vi "Factory.vi"(8 "error in":errorcluster, 10 "Class name":string) -> (0 "error out":errorcluster, 3 "Read Config out":refnum<class "Read Config File.lvclass">)   [LabVIEW 2025, in "Config Library.lvlib" / "Read Config File.lvclass"]
uses:
  Read Config File.lvclass
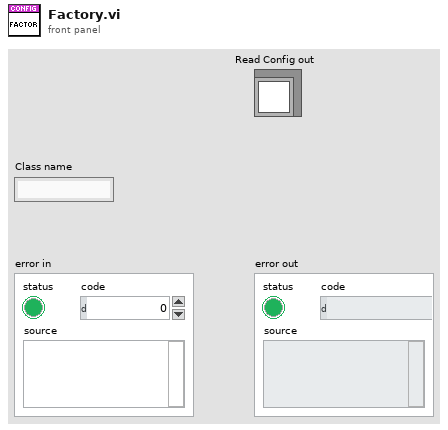
[diagram p1: front panel]
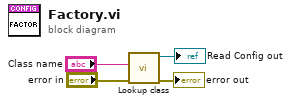
[diagram p0: block diagram]
diagram:
  n1 = call "Lookup class.vi"("error in"="error in", "Class name"="Class name") -> ("error out"=→"error out":errorcluster, "Read Config out"=→"Read Config out":refnum<class "Read Config File.lvclass">)  [unwired: 8 in]
